vi "Parse Bitfile Registers.vi"(6 "IP Classes":refnum<class "Engine Simulation IP.lvclass">[](array[class]), 8 "error in (no error)":errorcluster, 11 "bitfile":path) -> (0 "error out":errorcluster, 1 "EST version":T1, 2 "reg LUT":variant, 3 "EST version string":string)   [LabVIEW 2013, in "Engine Simulation Session.lvclass"]
uses:
  Engine Simulation Session.lvclass
  Bitfile Major Version.ctl
  Engine Simulation IP.lvclass
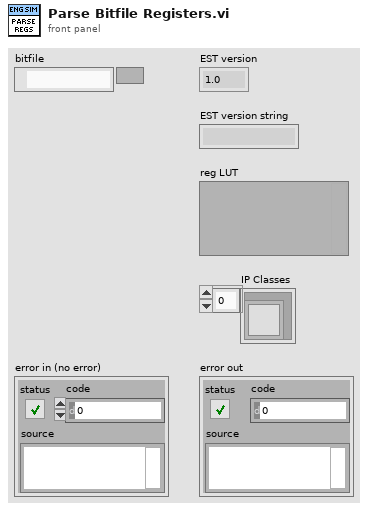
[diagram p1: front panel]
types:
  T1 = typedef "Engine Simulation Session.lvclass/Bitfile Major Version.ctl" = enum16{"1.0", "1.1", "1.2", "1.3"}
  T2 = typedef "niFpgaBitfileStructure_VI.ctl" = cluster{"Name":string, "RegisterMap":T3[], "Icon":T8}
  T3 = typedef "nirviControlStructure.ctl" = cluster{"Name":string, "Hidden":bool, "Indicator":bool, "Flattened Type":string, "Grouping":cluster{"Grouped":bool, "Member Names":string[], "Member IDs":u32[]}, "Address":u32, "Size":u32, "Class":u32, "Internal":bool, "Typedef":T4, "ID":u32, "Bidirectional":bool, "Synchronous":bool, "Mechanical Action":T5, "Sub Controls":T6[], "Access May Timeout":bool, "Register Node":bool}
  T4 = typedef "nirviTypdefDescription.ctl" = cluster{"Typedef":bool, "Path":path}
  T5 = typedef "nirviMechanicalAction.ctl" = enum8{"Switch When Pressed", "Switch When Released", "Switch Until Released", "Latch When Pressed", "Latch When Released", "Latch Until Released"}
  T6 = typedef "nirviSubControlStructure.ctl" = cluster{"Name":string, "flattened Type":string, "Cluster Information":T7, "Typedef":T4}
  T7 = typedef "nirviClusterElementControl.ctl" = cluster{"Name Hierarchy":string[], "Item Order":u32[]}
  T8 = typedef "imagedata.ctl" = cluster{"image type":i32, "image depth":i32, "image":u8[], "mask":u8[], "colors":u32[], "Rectangle":cluster{"left":i16, "top":i16, "right":i16, "bottom":i16}}
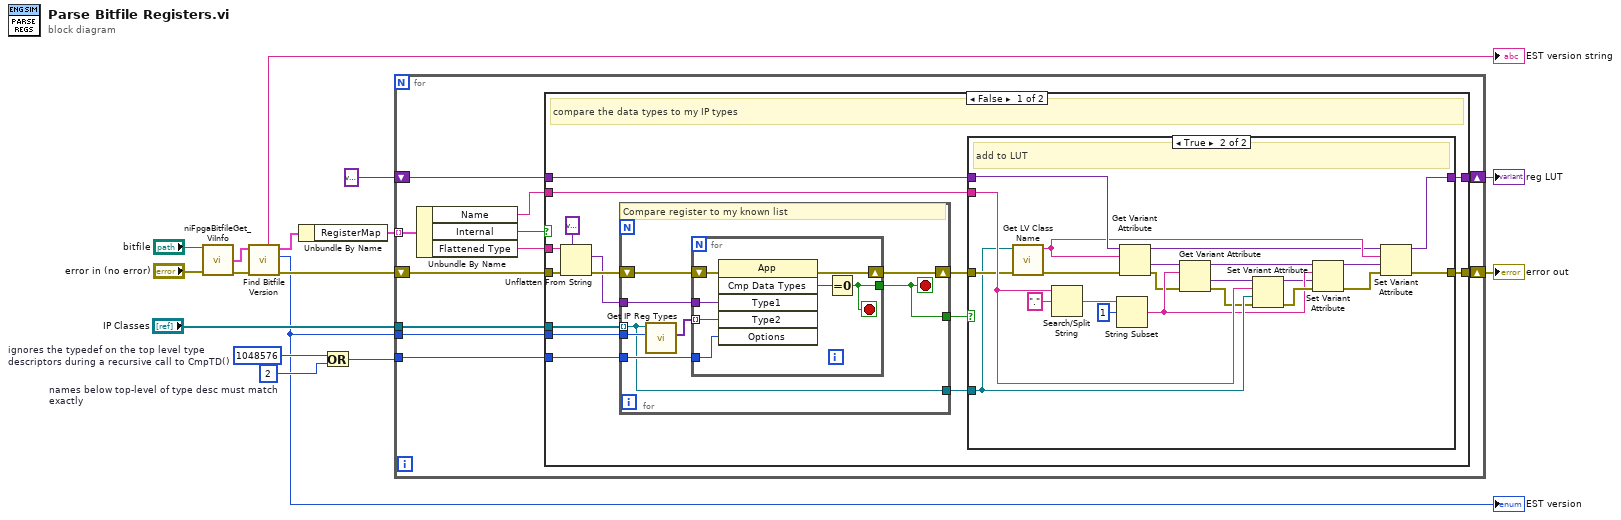
[diagram p0: block diagram]
diagram:
  w5 = 2  # names below top-level of type desc must match exactly
  w4 = 1048576  # ignores the typedef on the top level type descriptors during a recursive call to CmpTD()
  n1 = call <vilib>:"niFpgaBitfileGet_ViInfo.vi"("bitfile path"="bitfile", "error in (no error)"="error in (no error)") -> ("vi info"=w7:T2, "error out"=w3:errorcluster)  [unwired: 1 in, 11 out]
  n2 = call "Find Bitfile Version.vi"("error in (no error)"=w3, "vi info"=w7) -> ("error out"=w6:errorcluster, "EST version enum"=w1:T1, "vi info dup"=w8:T2, "EST version string"=→"EST version string":string)  [unwired: 5 in, 1 out]
  "EST version" <- w1
  n3 = Unbundle By Name(w8) -> ("RegisterMap"=w13:T3[])
  n4 = Or(x=w4, y=w5) -> (x .or. y?=w14:i32)
  n5 = for {
    shift-right: [w27] -> w10
    shift-left: w6 -> [w24]
    tunnel: w13 -> [w26] mode=indexing
    tunnel: w14 -> [w21]
    shift-right: [w19] -> w11
    shift-left: variant ("Variant") -> [w20]
    tunnel: "IP Classes" -> [w18]
    tunnel: w1 -> [w17]
    n6 = Unbundle By Name(w26) -> ("Name"=w25:string, "Internal"=w22:bool, "Flattened Type"=w23:string)
    n7 = case shown="False" w22 {
      tunnel: [w34 w83] -> w27
      tunnel: w25 -> [w33 _]
      tunnel: w24 -> [w41 w83]
      tunnel: w23 -> [w39 _]
      tunnel: w21 -> [w37 _]
      tunnel: w20 -> [w36 w82]
      tunnel: [w35 w82] -> w19
      tunnel: w18 -> [w30 _]
      tunnel: w17 -> [w29 _]
      frame False {
        # "compare the data types to my IP types"
        n8 = Unflatten From String(type=variant ("Variant"), binary string=w39, error in (no error)=w41) -> (value=w38:variant, error out=w42:errorcluster)  [unwired: 3 out]
        n9 = for {
          shift-right: [w73] -> w31
          shift-left: w42 -> [w74]
          tunnel: w38 -> [w72]
          tunnel: [w68] -> w32
          tunnel: w37 -> [w71]
          tunnel: w30 -> [w67] mode=indexing
          tunnel: w29 -> [w70]
          tunnel: [w67] -> w28
          stop <- w68 stop-if-true
          # "Compare register to my known list"
          n10 = call-dynamic "Get IP Reg Types.vi"("Version"=w70, "Engine Simulation IP in"=w67) -> ("IP Regs"=w69:variant[])  [unwired: 8 in, 1 out]
          n11 = for {
            tunnel: w72 -> [w79]
            tunnel: w69 -> [w78] mode=indexing
            tunnel: w71 -> [w77]
            shift-right: [w80] -> w73
            shift-left: w74 -> [w81]
            tunnel: [w75] -> w68
            stop <- w75 stop-if-true
            n12 = invoke class="App" method="Cmp Data Types"(error in=w81, "Type1"=w79, "Type2"=w78, "Options"=w77) -> (error out=w80:errorcluster, "Compare Data Types"=w76:i32)  [unwired: 2 in, 4 out]
            n13 = Equal To 0?(x=w76) -> (x = 0?=w75:bool)
          }
        }
        n14 = case shown="True" w32 {
          tunnel: w28 -> [_ w58]
          tunnel: w36 -> [w43 w63]
          tunnel: [w43 w61] -> w35
          tunnel: w33 -> [_ w64]
          tunnel: [w44 w62] -> w34
          tunnel: w31 -> [w44 w60]
          frame False {
          }
          frame True {
            # "add to LUT"
            n15 = call <vilib>:"Get LV Class Name.vi"("error in (no error)"=w60, "object"=w58) -> ("error out"=w59:errorcluster, "class name"=w57:string)  [unwired: 8 in]
            n16 = Search/Split String(string=w64, search string/char (-)=".") -> (match + rest of string=w65:string)  [unwired: 1 in, 2 out]
            n17 = String Subset(string=w65, offset (0)=1) -> (substring=w52:string)  [unwired: 1 in]
            n18 = Get Variant Attribute(Variant=w63, name=w57, error in=w59) -> (duplicate Variant=w46:variant, value=w47:variant, error out=w48:errorcluster)  [unwired: 1 in, 1 out]
            n19 = Get Variant Attribute(Variant=w47, name=w52, error in=w48) -> (duplicate Variant=w50:variant, value=w54:variant, error out=w55:errorcluster)  [unwired: 1 in, 1 out]
            n20 = Set Variant Attribute(Variant=w54, name=w64, value=w58, error in=w55) -> (Variant out=w51:variant, error out=w53:errorcluster)  [unwired: 1 out]
            n21 = Set Variant Attribute(Variant=w50, name=w52, value=w51, error in=w53) -> (Variant out=w45:variant, error out=w49:errorcluster)  [unwired: 1 out]
            n22 = Set Variant Attribute(Variant=w46, name=w57, value=w45, error in=w49) -> (Variant out=w61:variant, error out=w62:errorcluster)  [unwired: 1 out]
          }
        }
      }
      frame True {
        # "avoid internal registers. They don't have a type and users didnt make them anyway"
      }
    }
  }
  "reg LUT" <- w11
  "error out" <- w10
